vi "Caller.vi"(0 "Divide in":refnum<class "Divide.lvclass">, 2 "DVR In":refnum<data-value>, 5 "Sub Panel":refnum<vi>, 7 "User Event Ref":refnum<user-event>, 11 "Error In":errorcluster) -> (4 "Divide out":refnum<class "Divide.lvclass">, 15 "Error Out":errorcluster)   [LabVIEW 2023, in "Divide.lvclass"]
doc: "The VI asynchronously calls the Operation UI method of the division operation."
uses:
  Divide.lvclass
  C:/Users/Ancy.Augustin/Downloads/LVOOPS DVR/LVOOPS DVR/Classes/Arithemtic Operation/Arithemetic Operation.lvclass
  Arithemtic Operation/Arithemetic Operation.lvclass
  Typedef/User Event Data.ctl
  Operation UI.vi
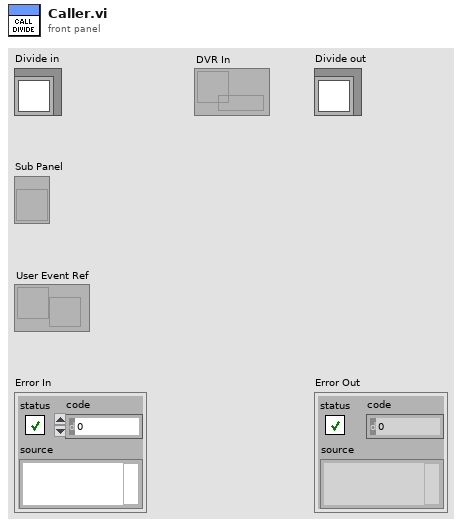
[diagram p1: front panel]
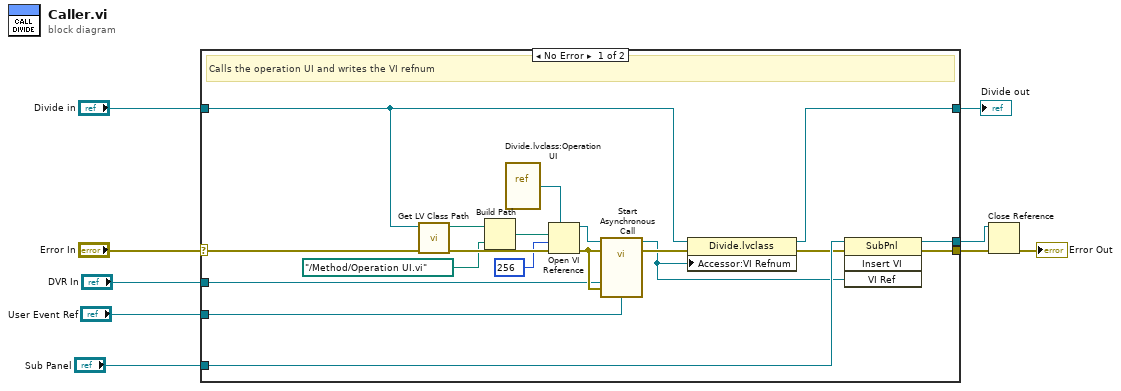
[diagram p0: block diagram]
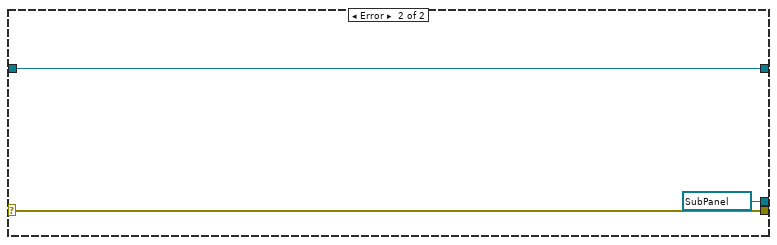
[diagram p2: hidden frame]
diagram:
  n1 = case shown="No Error" "Error In" {
    selector: "Error In" -> [w21 w31]
    tunnel: [w20 w31] -> w8
    tunnel: [w16 w30] -> w6
    tunnel: "Divide in" -> [w14 w30]
    tunnel: "Sub Panel" -> [w19 _]
    tunnel: [w15 refnum<vi> refnum ("Sub Panel")] -> w3
    tunnel: "DVR In" -> [w11 _]
    tunnel: "User Event Ref" -> [w10 _]
    frame No Error {
      # "Calls the operation UI and writes the VI refnum"
      n2 = call <vilib>:"Get LV Class Path.vi"("error in (no error)"=w21, "object"=w14) -> ("error out"=w28:errorcluster, "class path"=w27:path)  [unwired: 8 in]
      n3 = Build Path(base path=w27, name or relative path=path "../Method/Operation UI.vi") -> (appended path=w13:path)
      n4 = vi-ref "Divide.lvclass:Operation UI.vi"() -> (w22:refnum<vi>)
      n5 = Open VI Reference(type specifier VI Refnum (for type only)=w22, vi path=w13, options=256, error in (no error)=w28) -> (vi reference=w25:refnum<vi>, error out=w12:errorcluster)  [unwired: 2 in]
      n6 = call-by-ref "Start Asynchronous Call"(reference=w25, error in=w12, "DVR In"=w11, "Error In"=w12, "User Event Ref"=w10) -> (reference out=w17:refnum<vi>, error out=w24:errorcluster)  [unwired: 10 in, 3 out]
      n7 = property class="Divide.lvclass"(reference=w14, error in=w24, "Accessor:VI Refnum"=w17) -> (reference out=w16:refnum<class "Divide.lvclass">, error out=w18:errorcluster)
      n8 = invoke on="Invoke Node" class="SubPnl" method="Insert VI"(reference=w19, error in=w18, "VI Ref"=w17) -> (reference out=w15:refnum<vi>, error out=w20:errorcluster)  [unwired: 1 in, 2 out]
    }
    frame Error {
    }
  }
  "Divide out" <- w6
  n9 = Close Reference(reference=w3, error in (no error)=w8) -> (error out=→"Error Out":errorcluster)
